vi "BRig_Host__Loop_Consumer_RunState__main__v2.vi"(0 "input_hDataQueue":refnum<queue>, 5 "input_errorDataQueue":errorcluster, 7 "input_dataPlot":u16[][](array[numeric]), 9 "input_dataTS":u16[][](array[numeric]), 11 "input_idx":i32[](array[numeric]), 12 "threshold_1":u16, 13 "threshold_2":u16) -> (3 "output_ExpStart":bool, 4 "output_hDataQueue":refnum<queue>, 6 "output_errorDataQueue":errorcluster, 8 "output_dataPlot":u16[][](array[numeric]), 10 "output_dataTS":u16[][](array[numeric]), 14 "output_updatePlot":bool, 15 "output_idx":i32[](array[numeric]))   [LabVIEW 2014]
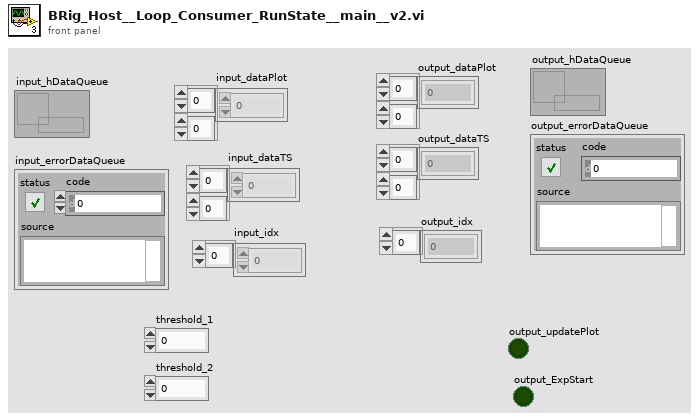
[diagram p1: front panel]
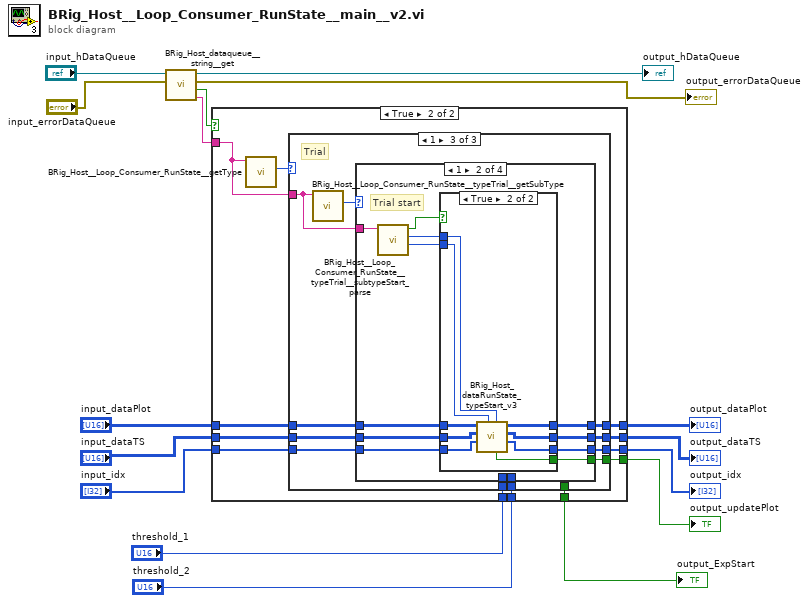
[diagram p0: block diagram]
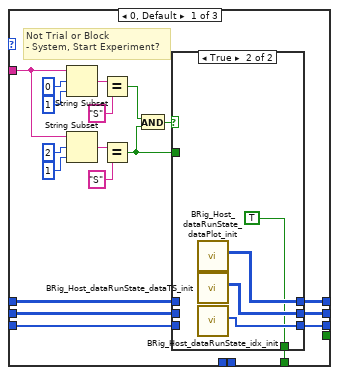
[diagram p3: hidden frame]
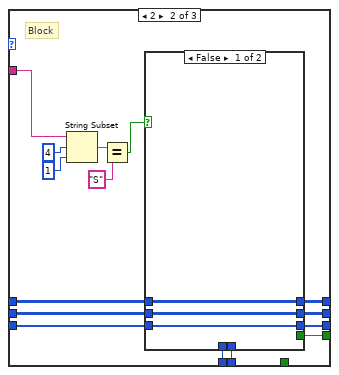
[diagram p5: hidden frame]
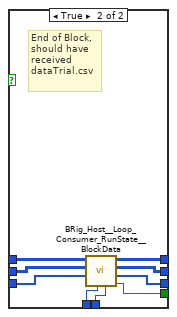
[diagram p6: hidden frame]
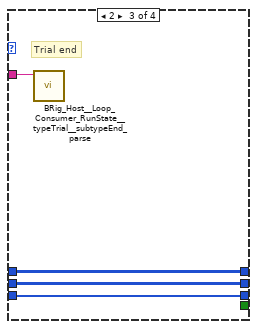
[diagram p9: hidden frame]
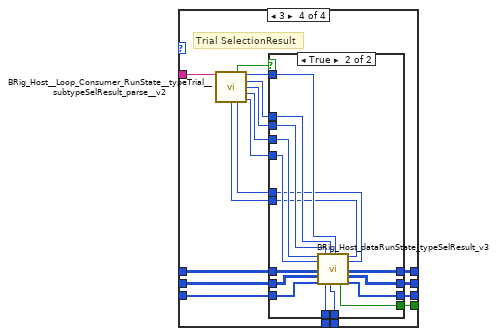
[diagram p10: hidden frame]
diagram:
  n1 = call "BRig_Host_dataqueue__string__get.vi"("input_errorDataQueue"="input_errorDataQueue", "input_hDataQueue"="input_hDataQueue") -> (0:"output_data"=w15:string, 1:"output_data"=w16:bool, "output_errorDataQueue"=→"output_errorDataQueue":errorcluster, "output_hDataQueue"=→"output_hDataQueue":refnum<queue>)  [unwired: 6 in]
  n2 = case shown="True" w16 {
    tunnel: w15 -> [_ w30]
    tunnel: "input_dataPlot" -> [w19 w29]
    tunnel: [w19 w28] -> w11
    tunnel: "input_dataTS" -> [w18 w27]
    tunnel: [w18 w26] -> w10
    tunnel: "input_idx" -> [w17 w25]
    tunnel: [w17 w24] -> w9
    tunnel: [_ w23] -> w8
    tunnel: "threshold_1" -> [_ w22]
    tunnel: "threshold_2" -> [_ w21]
    tunnel: [_ w20] -> w1
    frame False {
    }
    frame True {
      n3 = call "BRig_Host__Loop_Consumer_RunState__getType.vi"("input_strCmd"=w30) -> ("output_RunState_type"=w31:u8)  [unwired: 10 in]
      n4 = case shown="1" w31 {
        tunnel: w30 -> [w42 w68 w94]
        tunnel: w29 -> [w39 w67 w93]
        tunnel: [w38 w66 w92] -> w28
        tunnel: w27 -> [w37 w65 w91]
        tunnel: [w36 w64 w90] -> w26
        tunnel: w25 -> [w35 w63 w89]
        tunnel: [w34 w62 w88] -> w24
        tunnel: [_ w60 w87] -> w23
        tunnel: w22 -> [_ w59 w86]
        tunnel: w21 -> [_ w58 w85]
        tunnel: [w32 _ _] -> w20
        frame 0, Default {
          # "Not Trial or Block\n- System, Start Experiment?"
          n5 = String Subset(string=w42, offset (0)=0, length (rest)=1 ("offset (0)")) -> (substring=w49:string)
          n6 = String Subset(string=w42, offset (0)=2, length (rest)=1 ("offset (0)")) -> (substring=w45:string)
          n7 = Equal?(x=w49, y="S") -> (x = y?=w41:bool)
          n8 = Equal?(x=w45, y="S") -> (x = y?=w33:bool)
          n9 = And(x=w41, y=w33) -> (x .and. y?=w40:bool)
          n10 = case shown="True" w40 {
            tunnel: w39 -> [w53 _]
            tunnel: [w53 w55] -> w38
            tunnel: w37 -> [w52 _]
            tunnel: [w52 w56] -> w36
            tunnel: w35 -> [w51 _]
            tunnel: [w51 w57] -> w34
            tunnel: w33 -> [_ _]
            tunnel: [_ TRUE] -> w32
            frame False {
            }
            frame True {
              n11 = call "BRig_Host_dataRunState_dataPlot_init.vi"() -> ("output_dataPlot"=w55:u16[][])  [unwired: 11 in]
              n12 = call "BRig_Host_dataRunState_dataTS_init.vi"() -> ("output_dataTS"=w56:u16[][])  [unwired: 11 in]
              n13 = call "BRig_Host_dataRunState_idx_init.vi"() -> ("output_idx"=w57:i32[])  [unwired: 11 in]
            }
          }
        }
        frame 2 {
          # "Block"
          n14 = String Subset(string=w68, offset (0)=4, length (rest)=1 ("offset (0)")) -> (substring=w71:string)
          n15 = Equal?(x=w71, y="S") -> (x = y?=w61:bool)
          n16 = case shown="False" w61 {
            tunnel: w67 -> [w75 w84]
            tunnel: [w75 w83] -> w66
            tunnel: w65 -> [w74 w82]
            tunnel: [w74 w80] -> w64
            tunnel: w63 -> [w73 w81]
            tunnel: [w73 w79] -> w62
            tunnel: [_ w78] -> w60
            tunnel: w59 -> [_ w77]
            tunnel: w58 -> [_ w76]
            frame False {
            }
            frame True {
              # "End of Block,\nshould have\nreceived\ndataTrial.csv"
              n17 = call "BRig_Host__Loop_Consumer_RunState__BlockData.vi"("threshold_2"=w76, "threshold_1"=w77, "input_idx"=w81, "input_dataTS"=w82, "input_dataPlot"=w84) -> ("output_newData"=w78:bool, "output_idx"=w79:i32[], "output_dataTS"=w80:u16[][], "output_dataPlot"=w83:u16[][])  [unwired: 3 in]
            }
          }
        }
        frame 1 {
          # "Trial"
          n18 = call "BRig_Host__Loop_Consumer_RunState__typeTrial__getSubType.vi"("input_strCmd"=w94) -> ("output_Trial_subtype"=w95:u8)  [unwired: 10 in]
          n19 = case shown="1" w95 {
            tunnel: w94 -> [_ w109 w125 w143]
            tunnel: w93 -> [w98 w105 w124 w137]
            tunnel: [w98 w100 w124 w136] -> w92
            tunnel: w91 -> [w97 w104 w123 w135]
            tunnel: [w97 w101 w123 w134] -> w90
            tunnel: w89 -> [w96 w103 w122 w133]
            tunnel: [w96 w102 w122 w132] -> w88
            tunnel: [_ w99 _ w131] -> w87
            tunnel: w86 -> [_ _ _ w130]
            tunnel: w85 -> [_ _ _ w129]
            frame 0, Default {
            }
            frame 1 {
              # "Trial start"
              n20 = call "BRig_Host__Loop_Consumer_RunState__typeTrial__subtypeStart_parse.vi"("input_strCmd"=w109) -> ("output_LorR"=w107:u16, "output_nTrial"=w108:u16, "output_Start"=w106:bool)  [unwired: 8 in]
              n21 = case shown="True" w106 {
                tunnel: w108 -> [_ w113]
                tunnel: w107 -> [_ w114]
                tunnel: w105 -> [w110 w121]
                tunnel: w104 -> [w111 w120]
                tunnel: w103 -> [w112 w119]
                tunnel: [w112 w115] -> w102
                tunnel: [w111 w116] -> w101
                tunnel: [w110 w117] -> w100
                tunnel: [_ w118] -> w99
                frame False {
                }
                frame True {
                  n22 = call "BRig_Host_dataRunState_typeStart_v3.vi"("input_nTrial"=w113, "input_LorR"=w114, "input_idx"=w119, "input_dataTS"=w120, "input_dataPlot"=w121) -> ("output_idx"=w115:i32[], "output_dataTS"=w116:u16[][], "output_dataPlot"=w117:u16[][], "output_updatePlot"=w118:bool)  [unwired: 3 in]
                }
              }
            }
            frame 2 {
              # "Trial end"
              n23 = call "BRig_Host__Loop_Consumer_RunState__typeTrial__subtypeEnd_parse.vi"("input_strCmd"=w125) -> ()  [unwired: 10 in, 1 out]
            }
            frame 3 {
              # "Trial SelectionResult"
              n24 = call "BRig_Host__Loop_Consumer_RunState__typeTrial__subtypeSelResult_parse__v2.vi"("input_strCmd"=w143) -> ("output_selResult"=w128:bool, "output_nTrial"=w142:u16, "output_sSelection"=w141:u16, "output_tSelection"=w140:u16, "output_iReward_or_iError"=w139:u16, "output_trig_l2"=w126:u16, "output_trig_l1"=w127:u16, "output_LorR"=w138:u16)  [unwired: 7 in]
              n25 = case shown="True" w128 {
                tunnel: w142 -> [_ w151]
                tunnel: w141 -> [_ w152]
                tunnel: w140 -> [_ w153]
                tunnel: w139 -> [_ w154]
                tunnel: w138 -> [_ w155]
                tunnel: w137 -> [w146 w162]
                tunnel: [w146 w161] -> w136
                tunnel: w135 -> [w145 w157]
                tunnel: [w145 w160] -> w134
                tunnel: w133 -> [w144 w156]
                tunnel: [w144 w159] -> w132
                tunnel: [_ w158] -> w131
                tunnel: w130 -> [_ w150]
                tunnel: w129 -> [_ w149]
                tunnel: w127 -> [_ w147]
                tunnel: w126 -> [_ w148]
                frame False {
                }
                frame True {
                  n26 = call "BRig_Host_dataRunState_typeSelResult_v3.vi"("input_iSelection"=w154, "input_LorR"=w155, "input_dataPlot"=w162, "input_dataTS"=w157, "input_idx"=w156, "input_tSelection"=w153, "input_threshold_1"=w150, "input_sSelection"=w152, "input_threshold_2"=w149, "input_nTrial"=w151, "input_trig_l2"=w148, "input_trig_l1"=w147) -> ("output_updatePlot"=w158:bool, "output_dataPlot"=w161:u16[][], "output_dataTS"=w160:u16[][], "output_idx"=w159:i32[])  [unwired: 4 in]
                }
              }
            }
          }
        }
      }
    }
  }
  "output_updatePlot" <- w8
  "output_dataPlot" <- w11
  "output_dataTS" <- w10
  "output_idx" <- w9
  "output_ExpStart" <- w1
